vi "Write Element of Trigger Source.vi"(8 "error in (no error)":errorcluster, 9 "source (Immediate)":i32(ring) items=["Immediate", "External", "Software", "TTL0", "TTL1", "TTL2", "TTL3", "TTL4", "TTL5", "TTL6", "TTL7", "ECL0", "ECL1", "PXI Star", "RTSI 0", "RTSI 1", "RTSI 2", "RTSI 3", "RTSI 4", "RTSI 5", "RTSI 6"], 10 "index":i32, 11 "CS++DCPwrChannelData in":refnum<class "CS++DCPwrChannelData.lvclass">) -> (0 "error out":errorcluster, 3 "CS++DCPwrChannelData out":refnum<class "CS++DCPwrChannelData.lvclass">)   [LabVIEW 2013, in "CS++DCPwrGui.lvlib" / "CS++DCPwrChannelData.lvclass"]
uses:
  CS++DCPwrChannelData.lvclass
  CS++DCPwrChannelData.lvclass/CS++DCPwrChannelData.ctl
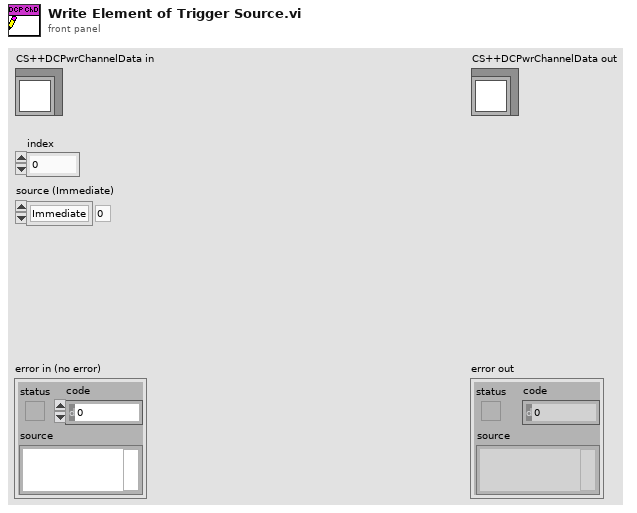
[diagram p1: front panel]
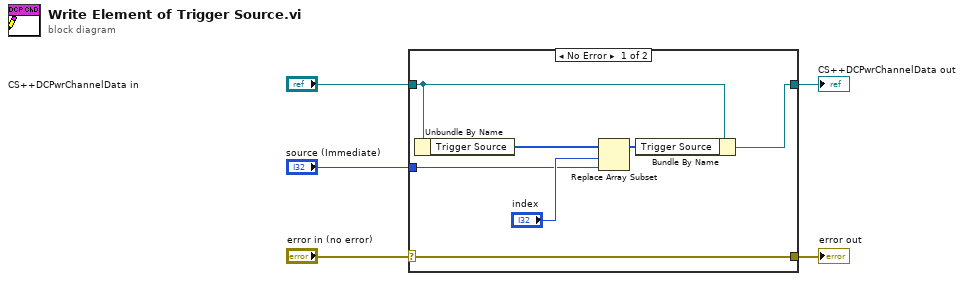
[diagram p0: block diagram]
diagram:
  n1 = case shown="No Error" "error in (no error)" {
    selector: "error in (no error)" -> [w12 w13]
    tunnel: [w12 w13] -> w4
    tunnel: [w11 w14] -> w2
    tunnel: "CS++DCPwrChannelData in" -> [w10 w14]
    tunnel: "source (Immediate)" -> [w6 _]
    frame No Error {
      n2 = Unbundle By Name(w10) -> ("Trigger Source"=w9:i32[])
      n3 = Replace Array Subset(array=w9, new element=w6, index="index") -> (w8:i32[])
      n4 = Bundle By Name(cluster=w10, "Trigger Source"=w8) -> (w11:refnum<class "CS++DCPwrChannelData.lvclass">)
    }
    frame Error {
    }
  }
  "error out" <- w4
  "CS++DCPwrChannelData out" <- w2
